vi "programa4.vi"() -> ()   [LabVIEW 2011]
panel:
  out "Alarma de Calentamiento":bool
  out "Temperatura":dbl(slide) scale=0.0..100.0
  out "Cambio":string
  out "Cuarta":bool
  out "Tercera":bool
  out "Segunda":bool
  out "Primera":bool
  out "Velocidad":i32(knob) scale=0.0..180.0
  # "Si la temperatura es mayor a\n75 y la velocidad mayor a \n120 encender alarma de \ncalentamiento."
  # "Elaborar un programa donde se genere la velocidad\nentre 1-180, luego de acuerdo a la velocidad que se \nalncance encender en que cambio se encuentra y escribir \nen el string indicator el cambio.\n\n1-40     primera\n41-60   segunda\n61-80   tercera\n81-180 cuarta"
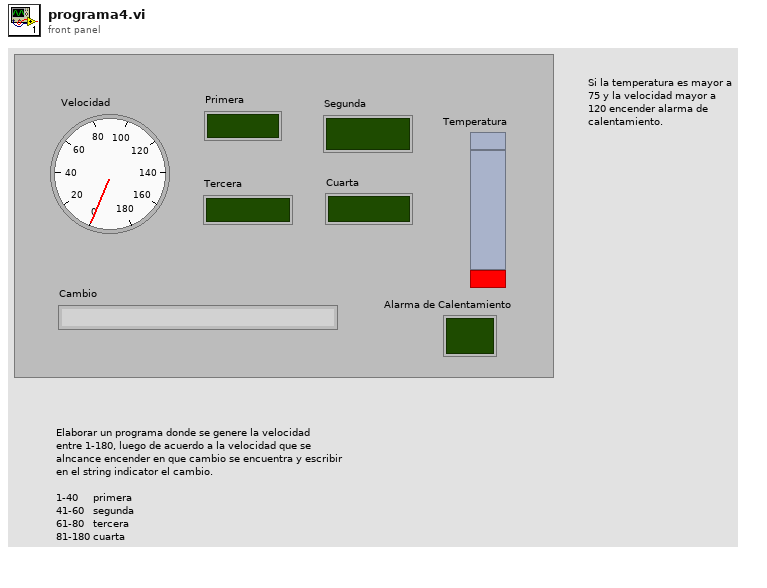
[diagram p1: front panel]
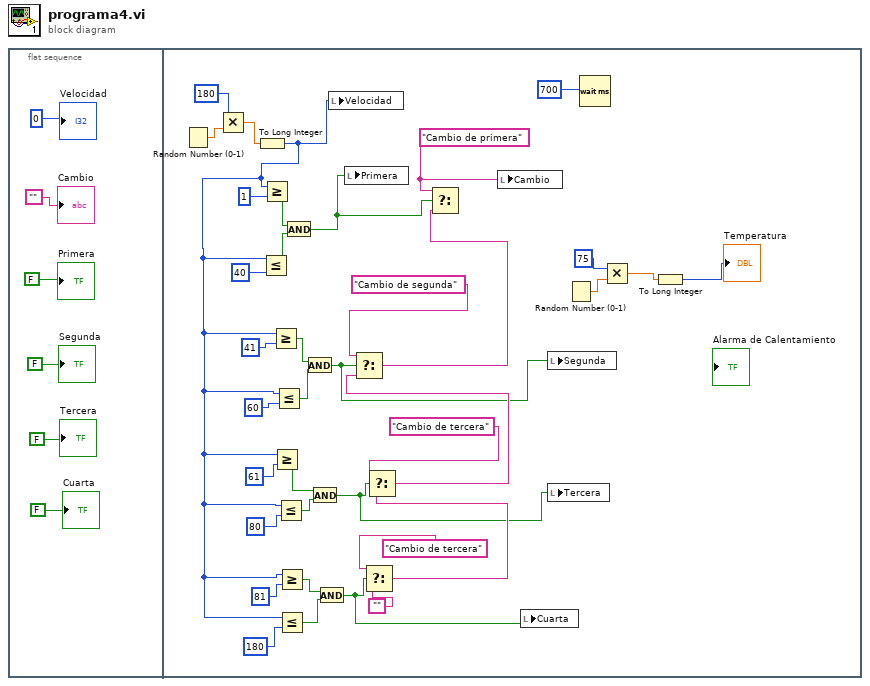
[diagram p0: block diagram]
diagram:
  n1 = flat-sequence {
    frame #0 {
      "Velocidad" <- 0
      "Primera" <- FALSE
      "Segunda" <- FALSE
      "Tercera" <- FALSE
      "Cuarta" <- FALSE
      "Cambio" <- ""
    }
    frame #1 {
      w35 = "Cambio de primera" ("Cambio")
      n2 = Random Number (0-1)() -> (number: 0 to 1=w41:dbl)
      n3 = Multiply(x=180, y=w41) -> (x*y=w42:dbl)
      n4 = To Long Integer(number=w42) -> (32bit integer=w22:i32)
      n5 = Less Or Equal?(x=w22, y=40) -> (x <= y?=w37:bool)
      n6 = Greater Or Equal?(x=w22, y=1) -> (x >= y?=w38:bool)
      n7 = Greater Or Equal?(x=w22, y=41) -> (x >= y?=w32:bool)
      n8 = Greater Or Equal?(x=w22, y=61) -> (x >= y?=w26:bool)
      n9 = Less Or Equal?(x=w22, y=60) -> (x <= y?=w31:bool)
      n10 = Less Or Equal?(x=w22, y=80) -> (x <= y?=w25:bool)
      n11 = Greater Or Equal?(x=w22, y=81) -> (x >= y?=w19:bool)
      n12 = Less Or Equal?(x=w22, y=180) -> (x <= y?=w18:bool)
      n13 = And(x=w38, y=w37) -> (x .and. y?=w36:bool)
      n14 = And(x=w32, y=w31) -> (x .and. y?=w12:bool)
      n15 = And(x=w26, y=w25) -> (x .and. y?=w13:bool)
      n16 = And(x=w19, y=w18) -> (x .and. y?=w14:bool)
      n17 = local write "Velocidad"(w22) -> ()
      n18 = local write "Primera"(w36) -> ()
      n19 = Select(t="Cambio de tercera" ("Cambio"), s=w14, f="") -> (s? t:f=w16:string)
      n20 = Select(t="Cambio de tercera" ("Cambio"), s=w13, f=w16) -> (s? t:f=w23:string)
      n21 = Select(t="Cambio de segunda" ("Cambio"), s=w12, f=w23) -> (s? t:f=w29:string)
      n22 = Select(t=w35, s=w36, f=w29) -> ()  [unwired: 1 out]
      n23 = local write "Cambio"(w35) -> ()
      n24 = local write "Cuarta"(w14) -> ()
      n25 = local write "Segunda"(w12) -> ()
      n26 = local write "Tercera"(w13) -> ()
      n27 = Random Number (0-1)() -> (number: 0 to 1=w9:dbl)
      n28 = Wait (ms)(milliseconds to wait=700) -> ()  [unwired: 1 out]
      n29 = Multiply(x=75, y=w9) -> (x*y=w8:dbl)
      n30 = To Long Integer(number=w8) -> (32bit integer=→"Temperatura":i32)
    }
  }
